vi "FP to HEX.vi"() -> ()   [LabVIEW 2013]
panel:
  out "Final Accel Values 5":dbl[][](array[numeric])
  out "Final Accel Values 4":dbl[][](array[numeric])
  out "Final Accel Values 3":dbl[][](array[numeric])
  out "Final Accel Values 2":dbl[][](array[numeric])
  in  "Final Accel Values 1":fxp<+/-,64,32>[][](array[numeric])
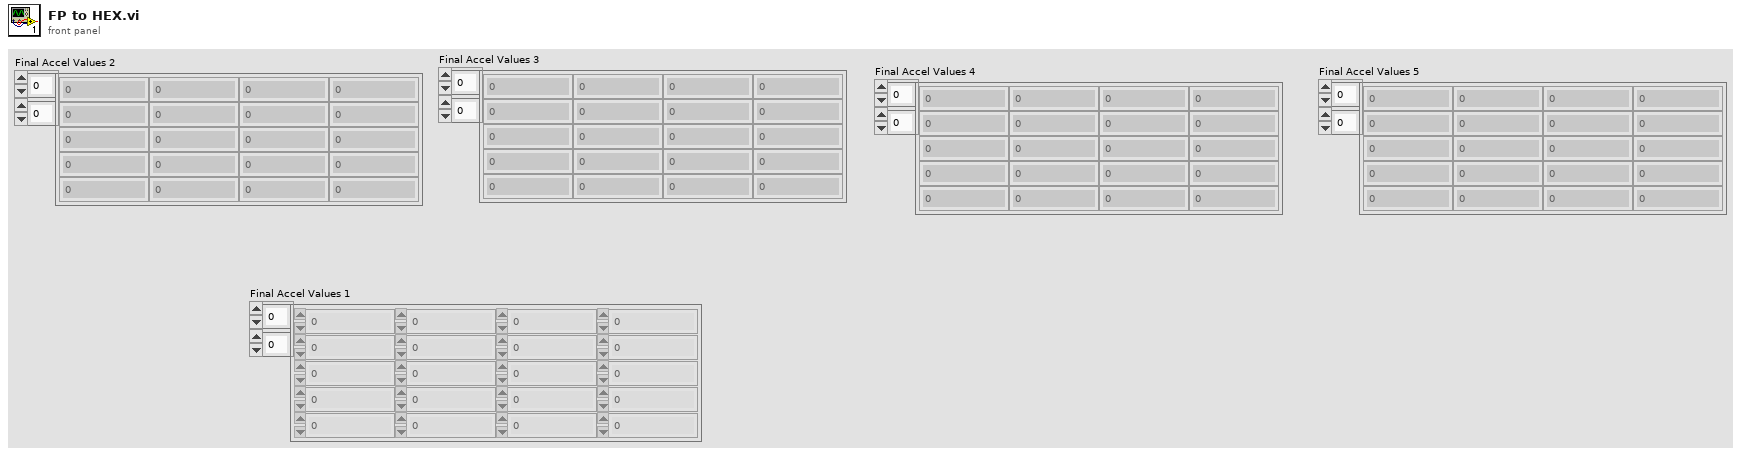
[diagram p1: front panel]
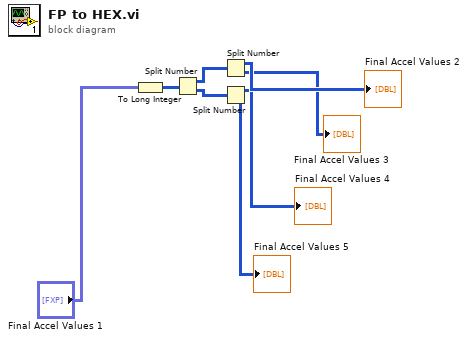
[diagram p0: block diagram]
diagram:
  n1 = To Long Integer(number="Final Accel Values 1") -> (32bit integer=w8:i32[][])
  n2 = Split Number(x=w8) -> (hi(x)=w7:u16[][], lo(x)=w6:u16[][])
  n3 = Split Number(x=w7) -> (hi(x)=→"Final Accel Values 2":u8[][], lo(x)=→"Final Accel Values 3":u8[][])
  n4 = Split Number(x=w6) -> (hi(x)=→"Final Accel Values 4":u8[][], lo(x)=→"Final Accel Values 5":u8[][])
